vi "Sample rate change.vi"(7 "SlaveID":u8=1, 8 "error in (no error)":errorcluster, 9 "Sample Rate":u16=3200, 11 ".NET Refnum in":refnum<k24>) -> (0 "error out":errorcluster, 3 ".NET Refnum out":refnum<k24>)   [LabVIEW 2017]
uses:
  C:/Users/chrisjan/Desktop/NowWorking/ITRI/DLL/Modbus.dll
  DLL/Modbus.dll
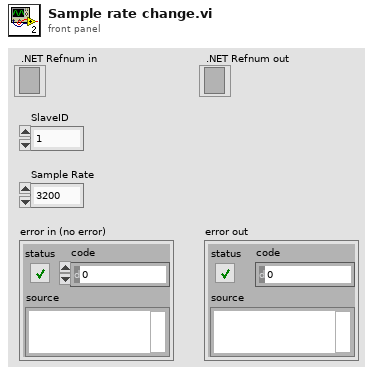
[diagram p1: front panel]
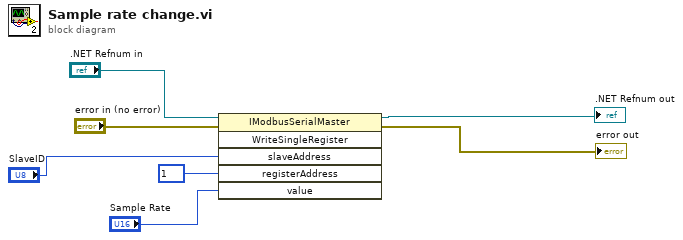
[diagram p0: block diagram]
diagram:
  n1 = invoke class="IModbusSerialMaster" method="WriteSingleRegister"(reference=".NET Refnum in", error in="error in (no error)", "slaveAddress"="SlaveID", "registerAddress"=u16 1 ("startAddress"), "value"="Sample Rate") -> (reference out=→".NET Refnum out":refnum<k24>, error out=→"error out":errorcluster)  [unwired: 1 in, 4 out]
